vi "construct.vi"(8 "error in (no error)":errorcluster, 11 "DAQ  in":refnum<class "DAQ .lvclass">) -> (0 "error out":errorcluster, 3 "DAQ  out":refnum<class "DAQ .lvclass">)   [LabVIEW 2026, in "Hardware.lvlib" / "DAQ .lvclass"]
uses:
  DAQ .lvclass
  C:/Users/E2013170/Documents/GitHub/Measurement-Utility-Reference/source/framework/Hardware/Hardware.lvclass
  config/DAQ Configuration.lvclass
  C:/Users/E2013170/Documents/GitHub/Measurement-Utility-Reference/source/framework/Hardware/HW Config/HW Configuration.lvclass
  framework/Hardware/Hardware.lvclass/Hardware.ctl
  framework/Hardware/Hardware.lvclass
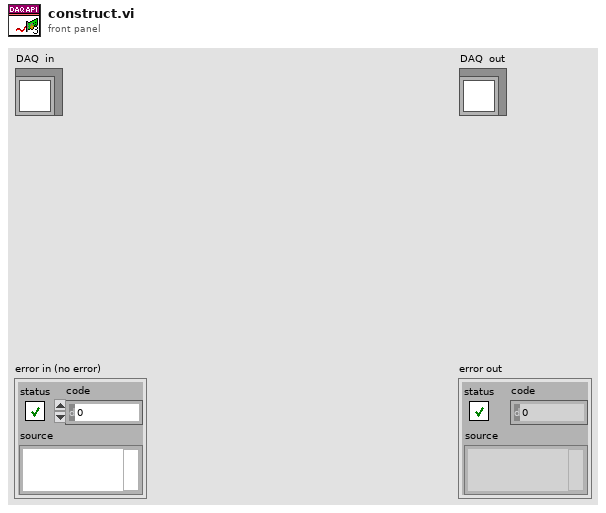
[diagram p1: front panel]
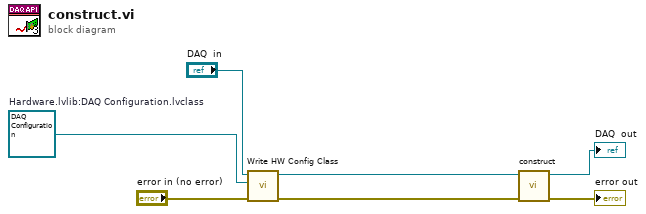
[diagram p0: block diagram]
diagram:
  w3 = refnum<class "DAQ Configuration.lvclass"> refnum  # Hardware.lvlib:DAQ Configuration.lvclass
  n1 = call "Write HW Config Class.vi"("error in (no error)"="error in (no error)", "Hardware.lvlib:HW Configuration.lvclass"=w3, "Hardware in"="DAQ  in") -> ("error out"=w1:errorcluster, "Hardware out"=w4:refnum<class "DAQ .lvclass">)  [unwired: 7 in]
  n2 = call-parent "construct.vi"("error in (no error)"=w1, "Hardware in"=w4) -> ("error out"=→"error out":errorcluster, "Hardware out"=→"DAQ  out":refnum<class "DAQ .lvclass">)  [unwired: 8 in]
